vi "Cross_spectra_and_phase.vi"(0 "U1":dbl[](array[numeric]) format="%.2f", 2 "U2":dbl[](array[numeric]) format="%.2f") -> (5 "U1 spectra":cluster{dbl, dbl, dbl[]}(graph), 6 "U2 spectra":cluster{dbl, dbl, dbl[]}(graph), 7 "U1 U2 coherence":cluster{dbl, dbl, "Coherence array":dbl[]}(graph), 8 "U1 U2 phase":cluster{dbl, dbl, "Phase array":dbl[]}(graph))   [LabVIEW 2010]
uses:
  Globals/Meas_global.vi
  <vilib>/Analysis/NI_AALBase.lvlib
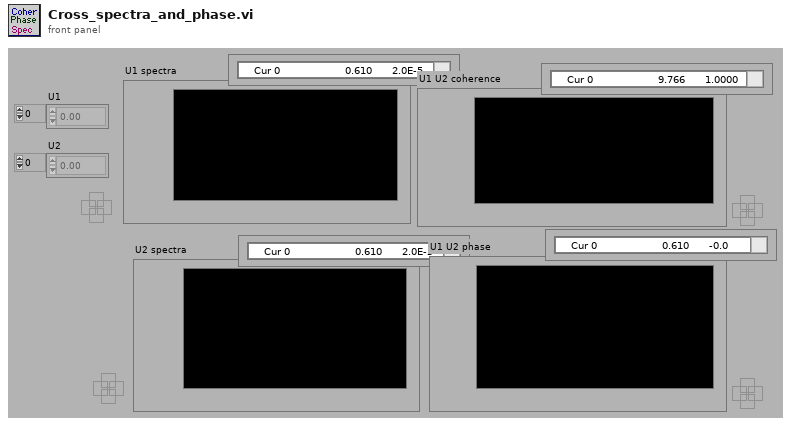
[diagram p1: front panel]
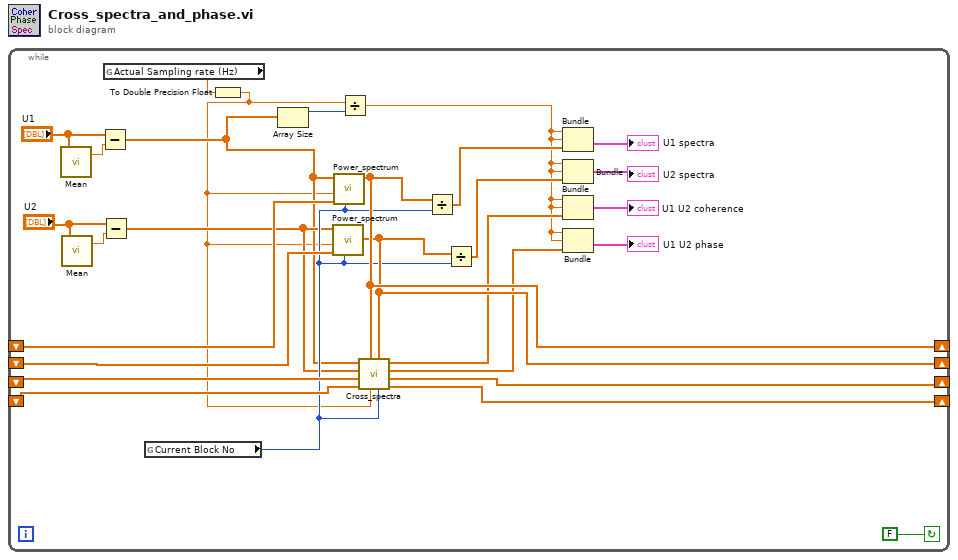
[diagram p0: block diagram]
diagram:
  n1 = while {
    shift-left: _ -> [w25]
    shift-right: [w23] -> _
    shift-left: _ -> [w26]
    shift-right: [w24] -> _
    shift-left: _ -> [w27]
    shift-right: [w21] -> _
    shift-left: _ -> [w28]
    shift-right: [w22] -> _
    stop <- FALSE continue-if-true
    n2 = call <vilib>:"Mean.vi"("X"="U1") -> ("mean"=w8:dbl)  [unwired: 1 out]
    n3 = call <vilib>:"Mean.vi"("X"="U2") -> ("mean"=w7:dbl)  [unwired: 1 out]
    n4 = Subtract(x="U1", y=w8) -> (x-y=w3:dbl[])
    n5 = Subtract(x="U2", y=w7) -> (x-y=w4:dbl[])
    n6 = global read "Meas_global.vi" "Actual Sampling rate (Hz)"() -> (w2:dbl)
    n7 = global read "Meas_global.vi" "Current Block No"() -> (w13:i32)
    n8 = To Double Precision Float(number=w2) -> (double precision float=w1:dbl)
    n9 = Array Size(array=w3) -> (size(s)=w14:i32)
    n10 = call "Power_spectrum.vi"("U"=w4, "Sampling frequency"=w1, "Spectrum input array"=w27, "Block No"=w13) -> ("Spectrum output array"=w21:dbl[])  [unwired: 1 in, 1 out]
    n11 = call "Power_spectrum.vi"("U"=w3, "Sampling frequency"=w1, "Spectrum input array"=w28, "Block No"=w13) -> ("Spectrum output array"=w22:dbl[])  [unwired: 1 in, 1 out]
    n12 = Divide(x=w1, y=w14) -> (x/y=w15:dbl)
    n13 = call "Cross_spectra.vi"("block number"=w13, "S11 input array"=w21, "sampling frequency"=w1, "S22 input array"=w22, "Im(S12) input array"=w25, "Re(S12) input array"=w26, "U2"=w4, "U1"=w3) -> ("Im(S12) output array"=w23:dbl[], "Re(S12) output array"=w24:dbl[], "Phase array"=w16:dbl[], "Coherence array"=w17:dbl[])
    n14 = Divide(x=w22, y=w13) -> (x/y=w19:dbl[])
    n15 = Divide(x=w21, y=w13) -> (x/y=w18:dbl[])
    n16 = Bundle(w15, w15, w19) -> (→"U1 spectra":cluster{dbl, dbl, dbl[]})  [unwired: 1 out]
    n17 = Bundle(w15, w15, w18) -> (→"U2 spectra":cluster{dbl, dbl, dbl[]})  [unwired: 1 out]
    n18 = Bundle(w15, w15, "Coherence array"=w17) -> (→"U1 U2 coherence":cluster{dbl, dbl, "Coherence array":dbl[]})  [unwired: 1 out]
    n19 = Bundle(w15, w15, "Phase array"=w16) -> (→"U1 U2 phase":cluster{dbl, dbl, "Phase array":dbl[]})  [unwired: 1 out]
  }
